vi "Set Bold.vi"(8 "error in":errorcluster, 10 "Bold":bool, 11 "Font in":refnum<class "Font.lvclass">) -> (0 "error out":errorcluster, 3 "Font out":refnum<class "Font.lvclass">)   [LabVIEW 2023, in "SourceGrid.lvlib" / "Font.lvclass"]
uses:
  Font.lvclass
  Font.lvclass/Font.ctl
  System.Drawing
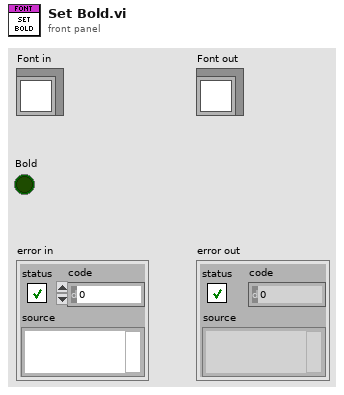
[diagram p1: front panel]
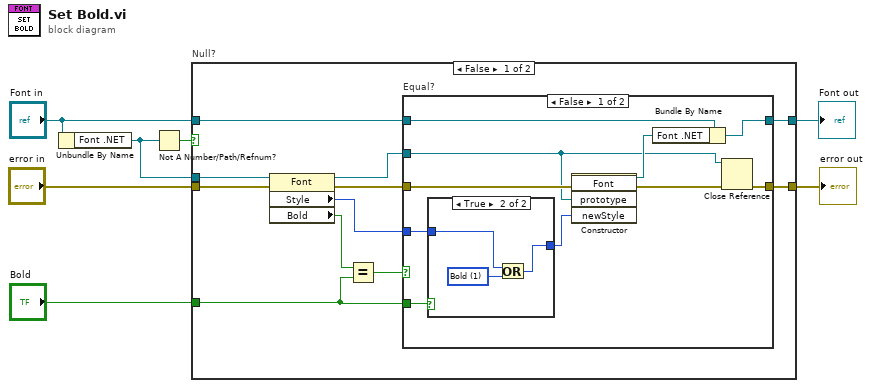
[diagram p0: block diagram]
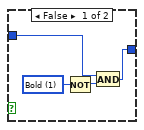
[diagram p2: hidden frame]
diagram:
  n1 = Unbundle By Name("Font in") -> ("Font .NET"=w1:refnum<k24>)
  n2 = Not A Number/Path/Refnum?(number/path/refnum=w1) -> (NaN/Path/Refnum?=w2:bool)
  n3 = case "Null?" shown="False" w2 {
    tunnel: w1 -> [w18 _]
    tunnel: "error in" -> [w17 w38]
    tunnel: "Bold" -> [w14 _]
    tunnel: [w11 w38] -> w5
    tunnel: "Font in" -> [w10 w39]
    tunnel: [w9 w39] -> w3
    frame False {
      n4 = property class="Font"(reference=w18, error in=w17) -> (reference out=w8:refnum<k24>, error out=w15:errorcluster, "Style"=w12:i32, "Bold"=w13:bool)
      n5 = Equal?(x=w13, y=w14) -> (x = y?=w16:bool)
      n6 = case "Equal?" shown="False" w16 {
        tunnel: w15 -> [w28 w37]
        tunnel: w14 -> [w22 _]
        tunnel: w12 -> [w21 _]
        tunnel: [w23 w37] -> w11
        tunnel: w10 -> [w27 w36]
        tunnel: [w25 w36] -> w9
        tunnel: w8 -> [w19 _]
        frame False {
          n7 = case shown="True" w22 {
            tunnel: w21 -> [w31 w34]
            tunnel: [w29 w33] -> w20
            frame False {
              w32 = 1 items=["Regular"=0, "Bold"=1, "Italic"=2, "Underline"=4, "Strikeout"=8] ("style")
              n8 = Not(x=w32) -> (.not. x?=w30:i32)
              n9 = And(x=w31, y=w30) -> (x .and. y?=w29:i32)
            }
            frame True {
              w35 = 1 items=["Regular"=0, "Bold"=1, "Italic"=2, "Underline"=4, "Strikeout"=8] ("style")
              n10 = Or(x=w34, y=w35) -> (x .or. y?=w33:i32)
            }
          }
          n11 = constructor class="Font" ("Constructor Font")(error in=w28, "prototype"=w19, "newStyle"=w20) -> (reference out=w26:refnum<k24>, error out=w24:errorcluster)  [unwired: 2 in, 3 out]
          n12 = Bundle By Name(cluster=w27, "Font .NET"=w26) -> (w25:refnum<class "Font.lvclass">)
          n13 = Close Reference(reference=w19, error in (no error)=w24) -> (error out=w23:errorcluster)
        }
        frame True {
        }
      }
    }
    frame True {
    }
  }
  "error out" <- w5
  "Font out" <- w3
